vi "Sub_Online_FEA_Main.vi"(8 "Bound Search":bool, 9 "Mode Count":i32=3 min=1 max=10 step=1, 10 "Eigenvalue Method":T2(ring), 11 "Experiment In":T1) -> (3 "Experiment Out":T1)   [LabVIEW 2021]
uses:
  <vilib>/Analysis/7linalg.llb/Eigenvalue and Vectors Output Option.ctl
  <vilib>/Analysis/baseanly.llb/Matrix Type of Inverse Matrix.ctl
  <vilib>/Analysis/7linalg.llb/Real Generalized Eigenvalues and Vectors.vi
  <vilib>/Analysis/7linalg.llb/Real Cholesky Factorization.vi
  <vilib>/Analysis/baseanly.llb/Full Cholesky Factorization.vi
  <vilib>/Analysis/baseanly.llb/Full Real Matrix Cholesky Factorization.vi
  <vilib>/Analysis/Matrix/Numeric/Conversions/Array To Matrix - RA2.vi
  <vilib>/Analysis/baseanly.llb/Real Inverse Matrix.vi
  <vilib>/Analysis/Matrix/Numeric/Multiply/Multiply - RM,RM.vi
  <vilib>/Analysis/7linalg.llb/Real Eigenvalues and Vectors.vi
  <vilib>/Analysis/Matrix/Numeric/Add/Add - RM,RM.vi
  <vilib>/Analysis/NI_AALPro.lvlib
  <vilib>/Analysis/Matrix/NI_Matrix.lvlib
  <vilib>/Analysis/NI_AALBase.lvlib
panel:
  out "Position estimate":dbl
  out "Pin estimate":i32
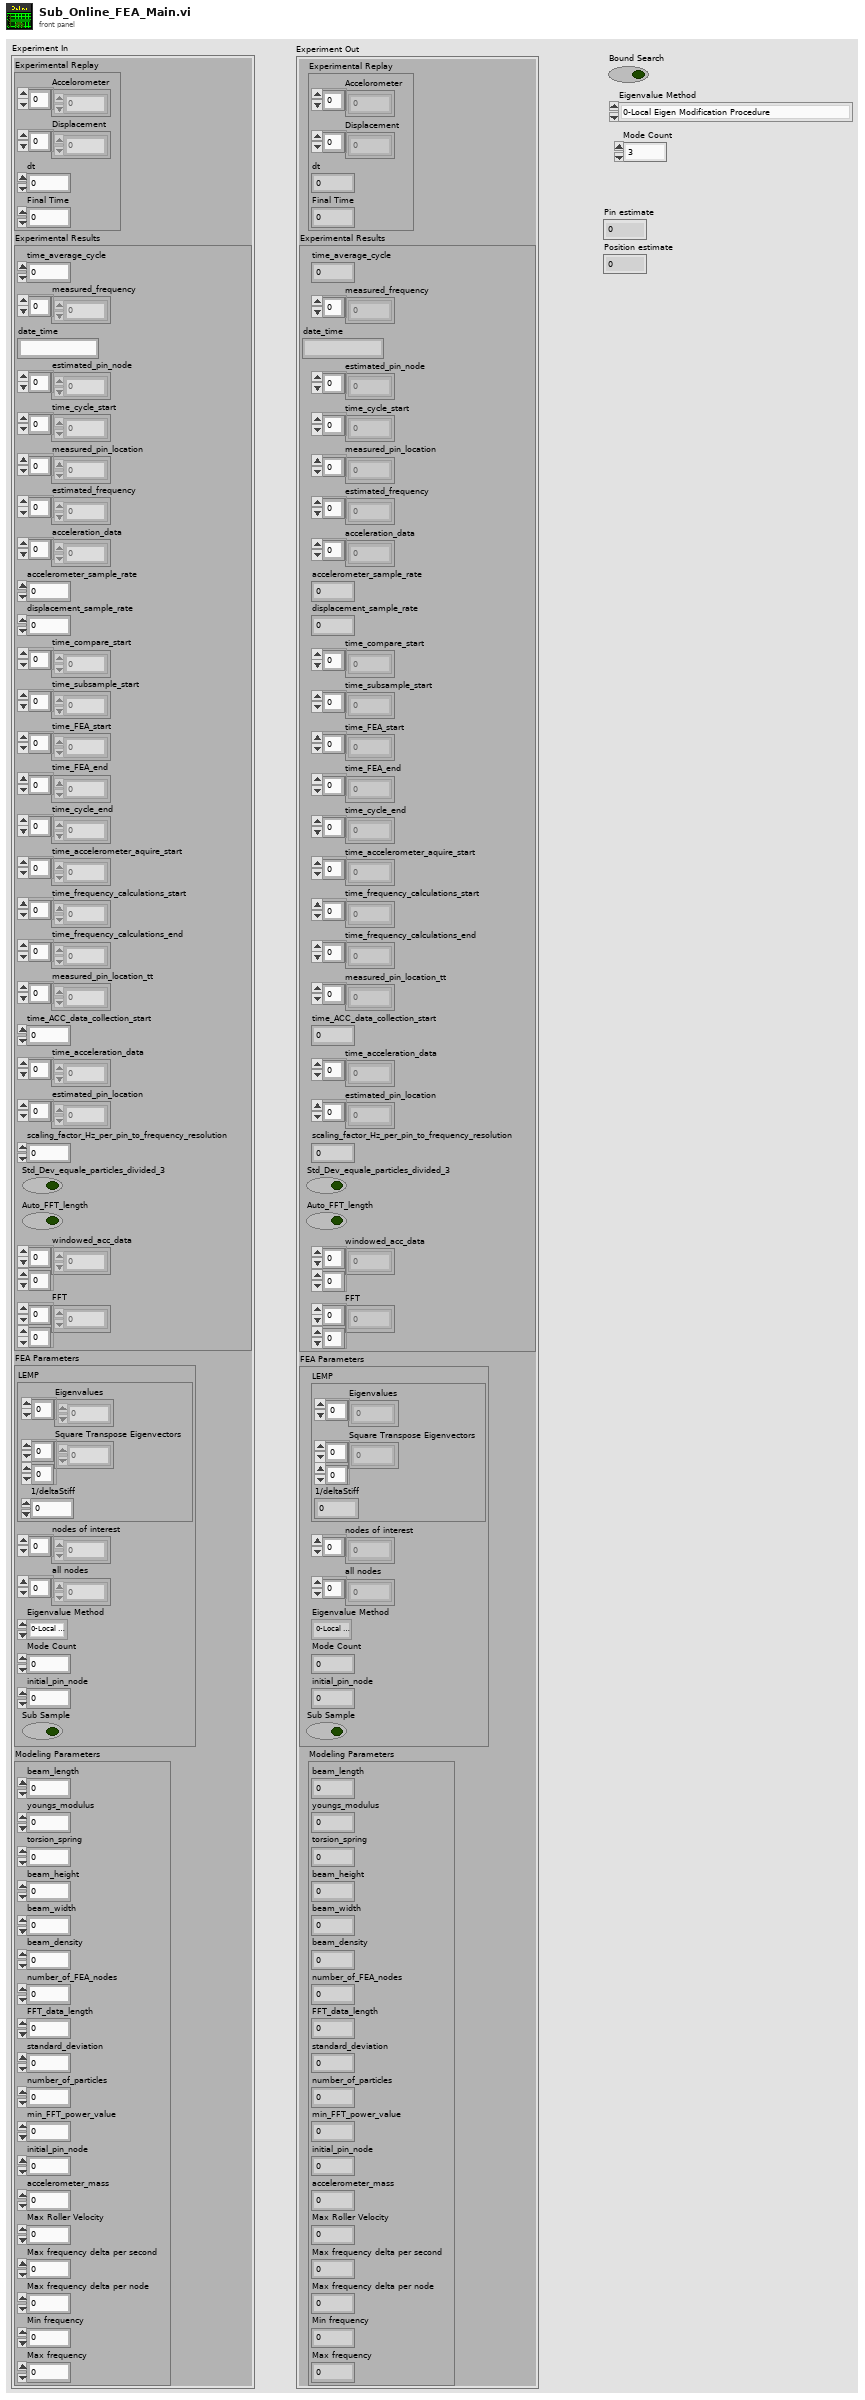
[diagram p1: front panel]
types:
  T1 = cluster{"Experimental Replay":cluster{"Accelorometer":dbl[], "Displacement":dbl[], "dt":dbl, "Final Time":dbl}, "Experimental Results":cluster{"time_average_cycle":dbl, "measured_frequency":dbl[], "date_time":string, "estimated_pin_node":i32[], "time_cycle_start":dbl[], "measured_pin_location":dbl[], "estimated_frequency":dbl[], "acceleration_data":dbl[], "accelerometer_sample_rate":dbl, "displacement_sample_rate":dbl, "time_compare_start":dbl[], "time_subsample_start":dbl[], "time_FEA_start":dbl[], "time_FEA_end":dbl[], "time_cycle_end":dbl[], "time_accelerometer_aquire_start":dbl[], "time_frequency_calculations_start":dbl[], "time_frequency_calculations_end":dbl[], "measured_pin_location_tt":dbl[], "time_ACC_data_collection_start":dbl, "time_acceleration_data":dbl[], "estimated_pin_location":dbl[], "scaling_factor_Hz_per_pin_to_frequency_resolution":dbl, "Std_Dev_equale_particles_divided_3":bool, "Auto_FFT_length":bool, "windowed_acc_data":dbl[][], "FFT":dbl[][]}, "FEA Parameters":cluster{"LEMP":cluster{"Eigenvalues":dbl[], "Square Transpose Eigenvectors":dbl[][], "1/deltaStiff":dbl}, "nodes of interest":i32[], "all nodes":i32[], "Eigenvalue Method":enum16{"0-Local Eigen Modification Procedure", "1-LabVIEW generalized eigenvalues", "2-LabVIEW M^-1K eigenvalues", "3-LabVIEW Cholesky Factorization", "4-Cholesky Factorization CPU SGL", "5-Cholesky Factorization CPU FXP", "6-Cholesky Factorization FPGA SGL", "7-Cholesky Factorization FPGA SGL SCL"}, "Mode Count":i32, "initial_pin_node":i32, "Sub Sample":bool}, "Modeling Parameters":cluster{"beam_length":dbl, "youngs_modulus":dbl, "torsion_spring":dbl, "beam_height":dbl, "beam_width":dbl, "beam_density":dbl, "number_of_FEA_nodes":i32, "FFT_data_length":i32, "standard_deviation":dbl, "number_of_particles":i32, "min_FFT_power_value":dbl, "initial_pin_node":i32, "accelerometer_mass":dbl, "Max Roller Velocity":dbl, "Max frequency delta per second":dbl, "Max frequency delta per node":dbl, "Min frequency":dbl, "Max frequency":dbl}}
  T2 = enum16{"0-Local Eigen Modification Procedure", "1-LabVIEW generalized eigenvalues", "2-LabVIEW M^-1K eigenvalues", "3-LabVIEW Cholesky Factorization", "4-Cholesky Factorization CPU SGL", "5-Cholesky Factorization CPU FXP", "6-Cholesky Factorization FPGA SGL", "7-Cholesky Factorization FPGA SGL SCL"}
  T3 = cluster{"LEMP":cluster{"Eigenvalues":dbl[], "Square Transpose Eigenvectors":dbl[][], "1/deltaStiff":dbl}, "nodes of interest":i32[], "all nodes":i32[], "Eigenvalue Method":enum16{"0-Local Eigen Modification Procedure", "1-LabVIEW generalized eigenvalues", "2-LabVIEW M^-1K eigenvalues", "3-LabVIEW Cholesky Factorization", "4-Cholesky Factorization CPU SGL", "5-Cholesky Factorization CPU FXP", "6-Cholesky Factorization FPGA SGL", "7-Cholesky Factorization FPGA SGL SCL"}, "Mode Count":i32, "initial_pin_node":i32, "Sub Sample":bool}
  T4 = cluster{"beam_length":dbl, "youngs_modulus":dbl, "torsion_spring":dbl, "beam_height":dbl, "beam_width":dbl, "beam_density":dbl, "number_of_FEA_nodes":i32, "FFT_data_length":i32, "standard_deviation":dbl, "number_of_particles":i32, "min_FFT_power_value":dbl, "initial_pin_node":i32, "accelerometer_mass":dbl, "Max Roller Velocity":dbl, "Max frequency delta per second":dbl, "Max frequency delta per node":dbl, "Min frequency":dbl, "Max frequency":dbl}
  T5 = cluster{"time_average_cycle":dbl, "measured_frequency":dbl[], "date_time":string, "estimated_pin_node":i32[], "time_cycle_start":dbl[], "measured_pin_location":dbl[], "estimated_frequency":dbl[], "acceleration_data":dbl[], "accelerometer_sample_rate":dbl, "displacement_sample_rate":dbl, "time_compare_start":dbl[], "time_subsample_start":dbl[], "time_FEA_start":dbl[], "time_FEA_end":dbl[], "time_cycle_end":dbl[], "time_accelerometer_aquire_start":dbl[], "time_frequency_calculations_start":dbl[], "time_frequency_calculations_end":dbl[], "measured_pin_location_tt":dbl[], "time_ACC_data_collection_start":dbl, "time_acceleration_data":dbl[], "estimated_pin_location":dbl[], "scaling_factor_Hz_per_pin_to_frequency_resolution":dbl, "Std_Dev_equale_particles_divided_3":bool, "Auto_FFT_length":bool, "windowed_acc_data":dbl[][], "FFT":dbl[][]}
  T6 = cluster{"Eigenvalues":dbl[], "Square Transpose Eigenvectors":dbl[][], "1/deltaStiff":dbl}
  T7 = typedef "NI_AALBase.lvlib/Matrix Type of Inverse Matrix.ctl" = enum32{"General", "Positive Definite", "Lower Triangular", "Upper Triangular"}
  T8 = typedef "NI_AALPro.lvlib/Eigenvalue and Vectors Output Option.ctl" = i32
  T9 = typedef "NI_Matrix.lvlib/RealMatrix.ctl" = dbl[][]
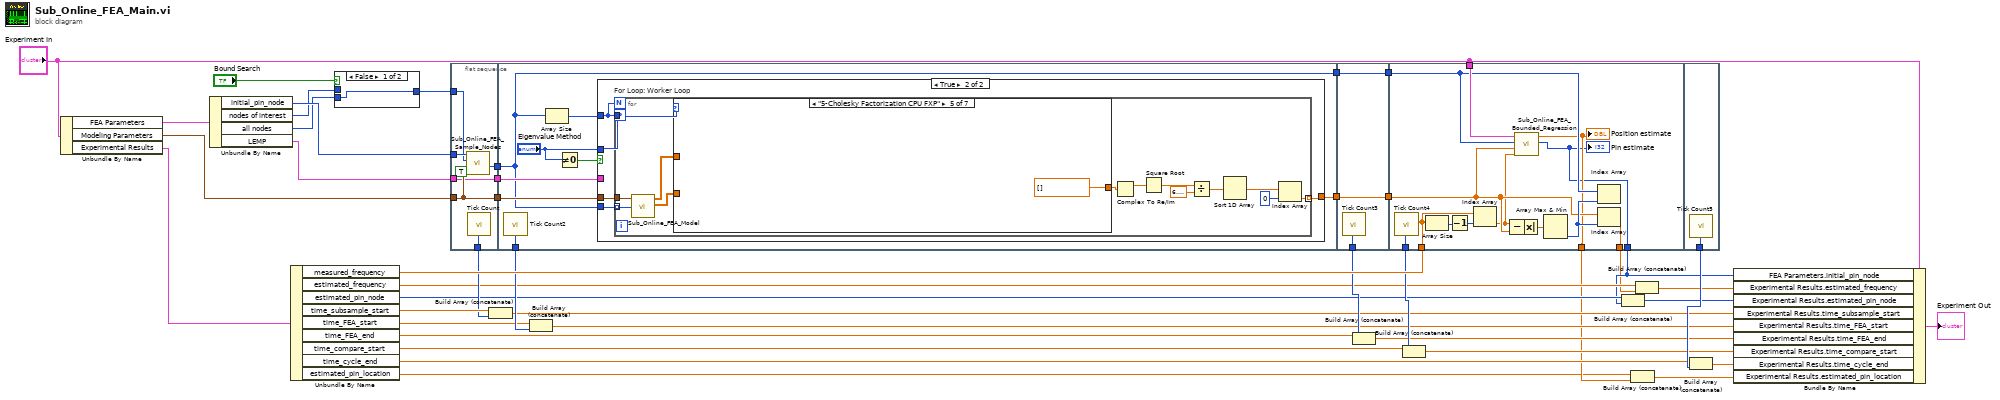
[diagram p0: block diagram]
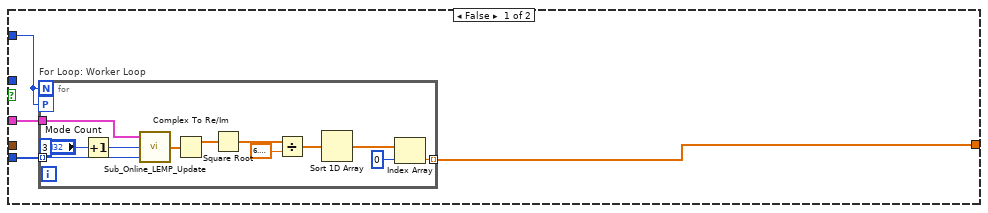
[diagram p3: hidden frame]
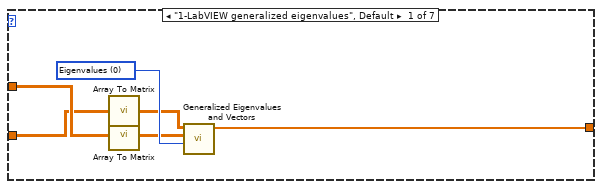
[diagram p4: hidden frame]
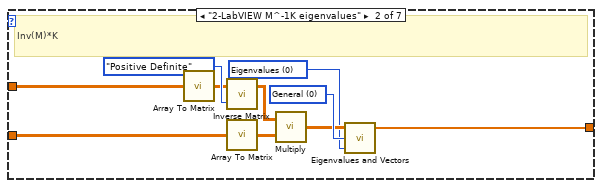
[diagram p5: hidden frame]
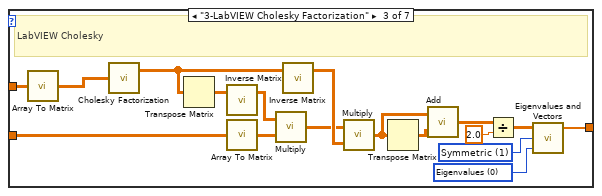
[diagram p6: hidden frame]
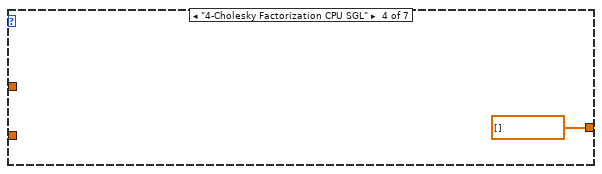
[diagram p7: hidden frame]
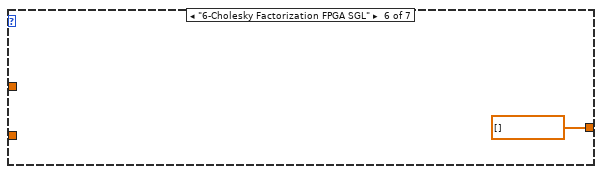
[diagram p8: hidden frame]
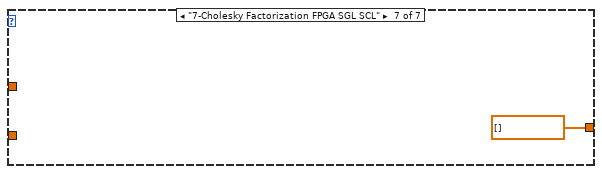
[diagram p9: hidden frame]
diagram:
  n1 = Unbundle By Name("Experiment In") -> ("FEA Parameters"=w16:T3, "Modeling Parameters"=w36:T4, "Experimental Results"=w17:T5)
  n2 = Unbundle By Name(w16) -> ("initial_pin_node"=w37:i32, "nodes of interest"=w35:i32[], "all nodes"=w34:i32[], "LEMP"=w33:T6)
  n3 = Unbundle By Name(w17) -> ("measured_frequency"=w31:dbl[], "estimated_frequency"=w18:dbl[], "estimated_pin_node"=w19:i32[], "time_subsample_start"=w28:dbl[], "time_FEA_start"=w25:dbl[], "time_FEA_end"=w24:dbl[], "time_compare_start"=w22:dbl[], "time_cycle_end"=w7:dbl[], "estimated_pin_location"=w2:dbl[])
  n4 = case shown="False" "Bound Search" {
    tunnel: w35 -> [_ w45]
    tunnel: w34 -> [w44 _]
    tunnel: [w44 w45] -> w38
    frame False {
    }
    frame True {
    }
  }
  n5 = flat-sequence {
    tunnel: w36 -> [w50]
    tunnel: [w50] -> w43
    tunnel: w37 -> [w52]
    tunnel: [w51] -> w27
    tunnel: w33 -> [w49]
    tunnel: [w49] -> w42
    tunnel: [w48] -> w41
    tunnel: w38 -> [w47]
    tunnel: w43 -> [w59]
    tunnel: [w60] -> w40
    tunnel: [w58] -> w26
    tunnel: w42 -> [w55]
    tunnel: w41 -> [w53]
    tunnel: [w53] -> w29
    tunnel: w40 -> [w134]
    tunnel: [w134] -> w39
    tunnel: [w133] -> w23
    tunnel: [w132] -> w30
    tunnel: w29 -> [w132]
    tunnel: w39 -> [w139]
    tunnel: [w145] -> w21
    tunnel: w31 -> [w144]
    tunnel: w30 -> [w140]
    tunnel: [w135] -> w14
    tunnel: "Experiment In" -> [w141]
    tunnel: [w137] -> w3
    tunnel: [w136] -> w1
    tunnel: [w149] -> w20
    frame #0 {
      n6 = call "Sub_Online_FEA_Sample_Nodes.vi"("include extremes"=TRUE, "Modeling Parameters"=w50, "FEA Nodes"=w47, "Initial Pin Location"=w52) -> ("Unique Samples"=w48:i32[])  [unwired: 5 in, 2 out]
      n7 = call "Tick Count"() -> ("Tick Count(uSec)"=w51:u32)
    }
    frame #1 {
      n8 = call "Tick Count2"() -> ("Tick Count(uSec)"=w58:u32)
      n9 = Array Size(array=w53) -> (size(s)=w54:i32)
      n10 = Not Equal To 0?(x="Eigenvalue Method") -> (x != 0?=w57:bool)
      n11 = case shown="True" w57 {
        tunnel: w53 -> [w63 w81]
        tunnel: [w62 w80] -> w60
        tunnel: w59 -> [_ w79]
        tunnel: w54 -> [w64 w78]
        tunnel: "Eigenvalue Method" -> [_ w77]
        tunnel: w55 -> [w61 _]
        frame False {
          n12 = for "For Loop: Worker Loop" {
            N: w64 -> [_]
            workers-P: w64 -> [_]
            tunnel: w63 -> [w66] mode=indexing
            tunnel: [w70] -> w62 mode=indexing
            tunnel: w61 -> [w65]
            (unwired) 3 ("Mode Count")
            n13 = Increment(x="Mode Count") -> (x+1=w67:i32)
            n14 = call "Sub_Online_LEMP_Update.vi"("Effected DOF"=w66, "Mode count"=w67, "LEMP"=w65) -> ("Updated Eigenvalues"=w69:dbl[])
            n15 = Complex To Re/Im ("Complex To Cartesian.vi")(x + iy=w69) -> (x=w76:dbl[])  [unwired: 1 out]
            n16 = Square Root ("Square Root.vi")(x=w76) -> (sqrt(x)=w75:dbl[])
            n17 = Divide(x=w75, y=6.283185307179586) -> (x/y=w71:dbl[])
            n18 = Sort 1D Array(array=w71) -> (sorted array=w73:dbl[])
            n19 = Index Array(array=w73, index=0) -> (element=w70:dbl)
          }
        }
        frame True {
          n20 = for "For Loop: Worker Loop" {
            N: w78 -> [_]
            tunnel: [w89] -> w80 mode=indexing
            tunnel: w81 -> [w86] mode=indexing
            tunnel: w79 -> [w82]
            workers-P: w78 -> [_]
            tunnel: w77 -> [w83]
            n21 = call "Sub_Online_FEA_Model.vi"("Pin Location"=w86, "Modeling Parameters"=w82) -> ("K Matrix"=w85:dbl[][], "M Matrix"=w84:dbl[][])  [unwired: 8 in]
            n22 = case shown="\"5-Cholesky Factorization CPU FXP\"" w83 {
              tunnel: w84 -> [w98 w104 w112 _ _ _ _]
              tunnel: w85 -> [w97 w102 w114 _ _ _ _]
              tunnel: [w99 w107 w115 cdb[] [] ("Eigenvalues") cdb[] [] ("Eigenvalues") cdb[] [] ("Eigenvalues") cdb[] [] ("Eigenvalues")] -> w87
              frame "1-LabVIEW generalized eigenvalues", Default {
                w100 = T8 0 items=["Eigenvalues", "Eigenvalues & Vectors"] ("output option")
                n23 = call-poly <vilib>:"Array To Matrix.vi"("Real 2D Array"=w97) -> ("Real Matrix"=w96:T9)
                n24 = call-poly <vilib>:"Array To Matrix.vi"("Real 2D Array"=w98) -> ("Real Matrix"=w95:T9)
                n25 = call-poly <vilib>:"Generalized Eigenvalues and Vectors.vi"("output option"=w100, "B"=w95, "A"=w96) -> ("Eigenvalues"=w99:cdb[])  [unwired: 3 in, 2 out]
              }
              frame "2-LabVIEW M^-1K eigenvalues" {
                w106 = T8 0 items=["Eigenvalues", "Eigenvalues & Vectors"] ("output option")
                w109 = 0 items=["General", "Symmetric"] ("matrix type")
                # "Inv(M)*K"
                n26 = call-poly <vilib>:"Array To Matrix.vi"("Real 2D Array"=w104) -> ("Real Matrix"=w103:T9)
                n27 = call-poly <vilib>:"Inverse Matrix.vi"("matrix type"=Matrix_Type_of_Inverse_Matrix."Positive Definite", "Input Matrix"=w103) -> ("Inverse Matrix"=w110:T9)  [unwired: 1 out]
                n28 = call-poly <vilib>:"Array To Matrix.vi"("Real 2D Array"=w102) -> ("Real Matrix"=w101:T9)
                n29 = call-poly <vilib>:"Multiply.vi"("Real Matrix B"=w101, "Real Matrix A"=w110) -> ("A * B"=w108:T9)
                n30 = call-poly <vilib>:"Eigenvalues and Vectors.vi"("output option"=w106, "matrix type"=w109, "Input Matrix"=w108) -> ("Eigenvalues"=w107:cdb[])  [unwired: 2 out]
              }
              frame "3-LabVIEW Cholesky Factorization" {
                w117 = T8 0 items=["Eigenvalues", "Eigenvalues & Vectors"] ("output option")
                w118 = 1 items=["General", "Symmetric"] ("matrix type")
                # "LabVIEW Cholesky"
                n31 = call-poly <vilib>:"Array To Matrix.vi"("Real 2D Array"=w112) -> ("Real Matrix"=w111:T9)
                n32 = call-poly <vilib>:"Cholesky Factorization.vi"("A"=w111) -> ("Cholesky"=w126:T9)  [unwired: 1 out]
                n33 = Transpose Matrix(1:w126) -> (0:w127:T9)
                n34 = call-poly <vilib>:"Inverse Matrix.vi"("Input Matrix"=w127) -> ("Inverse Matrix"=w125:T9)  [unwired: 1 in, 1 out]
                n35 = call-poly <vilib>:"Array To Matrix.vi"("Real 2D Array"=w114) -> ("Real Matrix"=w113:T9)
                n36 = call-poly <vilib>:"Multiply.vi"("Real Matrix B"=w113, "Real Matrix A"=w125) -> ("A * B"=w123:T9)
                n37 = call-poly <vilib>:"Inverse Matrix.vi"("Input Matrix"=w126) -> ("Inverse Matrix"=w124:T9)  [unwired: 1 in, 1 out]
                n38 = call-poly <vilib>:"Multiply.vi"("Real Matrix B"=w124, "Real Matrix A"=w123) -> ("A * B"=w122:T9)
                n39 = Transpose Matrix(1:w122) -> (0:w121:T9)
                n40 = call-poly <vilib>:"Add.vi"("Real Matrix B"=w121, "Real Matrix A"=w122) -> ("A + B"=w119:T9)
                n41 = Divide(x=w119, y=2.0) -> (x/y=w116:T9)
                n42 = call-poly <vilib>:"Eigenvalues and Vectors.vi"("output option"=w117, "matrix type"=w118, "Input Matrix"=w116) -> ("Eigenvalues"=w115:cdb[])  [unwired: 2 out]
              }
              frame "4-Cholesky Factorization CPU SGL" {
              }
              frame "5-Cholesky Factorization CPU FXP" {
              }
              frame "6-Cholesky Factorization FPGA SGL" {
              }
              frame "7-Cholesky Factorization FPGA SGL SCL" {
              }
            }
            n43 = Complex To Re/Im ("Complex To Cartesian.vi")(x + iy=w87) -> (x=w94:dbl[])  [unwired: 1 out]
            n44 = Square Root ("Square Root.vi")(x=w94) -> (sqrt(x)=w93:dbl[])
            n45 = Divide(x=w93, y=6.283185307179586) -> (x/y=w88:dbl[])
            n46 = Sort 1D Array(array=w88) -> (sorted array=w91:dbl[])
            n47 = Index Array(array=w91, index=0) -> (element=w89:dbl)
          }
        }
      }
    }
    frame #2 {
      n48 = call "Tick Count3"() -> ("Tick Count(uSec)"=w133:u32)
    }
    frame #3 {
      n49 = call "Tick Count4"() -> ("Tick Count(uSec)"=w145:u32)
      n50 = Array Size(array=w144) -> (size(s)=w142:i32)
      n51 = Decrement(x=w142) -> (x-1=w143:i32)
      n52 = Index Array(array=w144, index=w143) -> (element=w138:dbl)
      n53 = Subtract(x=w138, y=w139) -> (x-y=w148:dbl[])
      n54 = call "Sub_Online_FEA_Bounded_Regression.vi"("Measuerd Frequency"=w138, "Frequency"=w139, "Pin"=w140, "Experiment in"=w141) -> ("Pin estimate"=w135:i32, "Position estimate"=w137:dbl)  [unwired: 6 in]
      "Pin estimate" <- w135
      "Position estimate" <- w137
      n55 = Absolute Value(x=w148) -> (abs(x)=w146:dbl[])
      n56 = Array Max & Min(array=w146) -> (min index (indices)=w147:i32)  [unwired: 3 out]
      n57 = Index Array(array=w140, index=w147) -> ()  [unwired: 1 out]
      n58 = Index Array(array=w139, index=w147) -> (element=w136:dbl)
    }
    frame #4 {
      n59 = call "Tick Count5"() -> ("Tick Count(uSec)"=w149:u32)
    }
  }
  n60 = Build Array (concatenate)(w28, w27) -> (w11:dbl[])
  n61 = Build Array (concatenate)(w25, w26) -> (w10:dbl[])
  n62 = Build Array (concatenate)(w24, w23) -> (w9:dbl[])
  n63 = Build Array (concatenate)(w22, w21) -> (w8:dbl[])
  n64 = Build Array (concatenate)(w19, w14) -> (w12:i32[])
  n65 = Build Array (concatenate)(w2, w3) -> (w4:dbl[])
  n66 = Build Array (concatenate)(w18, w1) -> (w13:dbl[])
  n67 = Build Array (concatenate)(w7, w20) -> (w5:dbl[])
  n68 = Bundle By Name(cluster="Experiment In", "FEA Parameters.initial_pin_node"=w14, "Experimental Results.estimated_frequency"=w13, "Experimental Results.estimated_pin_node"=w12, "Experimental Results.time_subsample_start"=w11, "Experimental Results.time_FEA_start"=w10, "Experimental Results.time_FEA_end"=w9, "Experimental Results.time_compare_start"=w8, "Experimental Results.time_cycle_end"=w5, "Experimental Results.estimated_pin_location"=w4) -> (→"Experiment Out":T1)
